vi "Strip N level.vi"(10 "Level":i32, 11 "path in":path) -> (3 "path out":path)   [LabVIEW 2025]
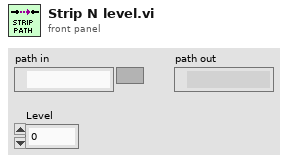
[diagram p1: front panel]
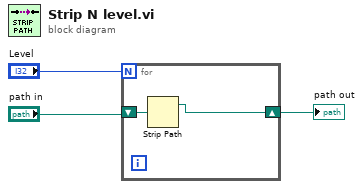
[diagram p0: block diagram]
diagram:
  n1 = for {
    N: "Level" -> [_]
    shift-right: [w4] -> w3
    shift-left: "path in" -> [w5]
    n2 = Strip Path(path=w5) -> (stripped path=w4:path)  [unwired: 1 out]
  }
  "path out" <- w3
